vi "FCI_Lip_Gap.vi"(0 "Image":T4(plugin-control), 1 "Calibrated Image":T4, 2 "Search Direction Ref ROI":u32=2, 3 "Ref ROI":T5 {"Contours"."Type" items=["No Selection", "Point", "Line", "Rectangle", "Oval", "Polygon", "Freehand Region", "Annulus", "Unused2", "Unused3", "Broken Line", "Freehand Line", "Rotated Rectangle"]}, 4 "Meas ROI 1":T5 {"Contours"."Type" items=["No Selection", "Point", "Line", "Rectangle", "Oval", "Polygon", "Freehand Region", "Annulus", "Unused2", "Unused3", "Broken Line", "Freehand Line", "Rotated Rectangle"]}, 5 "error in (no error)":errorcluster, 6 "Line Options Ref ROI":T8={"Number of Lines"=1, "Type"=enum."Best Edge Rake", "Min. Score"=10.0, "Max. Score"=1000.0, "Orientation"=0.0, "Angle Range"=45.0, "Angle Tolerance"=1.0, "Step Size"=5, "Min. SNR (db)"=0.0, "Min. Points (%)"=25.0, "Hough Iterations"=5} {"Min. Points (%)" min=0.0 max=100.0; "Min. SNR (db)" min=0.0; "Max. Score" min=0.0 max=1024.0; "Min. Score" min=0.0 max=1024.0 step=1.0}, 7 "Edge Options Ref ROI":T6={"Edge Polarity"=0, "Kernel Size"=3, "Width"=3, "Minimum Edge Strength"=40.0, "Interpolation Type"=enum."Zero Order", "Data Processing Method"=enum."Average"} {"Edge Polarity" items=["All Edges", "Rising Edges", "Falling Edges"]; "Minimum Edge Strength" format="%.2f"; "Width" step=2; "Kernel Size" step=2}, 8 "Edge Options ROI 1":T6={"Edge Polarity"=0, "Kernel Size"=3, "Width"=3, "Minimum Edge Strength"=50.0, "Interpolation Type"=enum."Zero Order", "Data Processing Method"=enum."Average"} {"Edge Polarity" items=["All Edges", "Rising Edges", "Falling Edges"]; "Minimum Edge Strength" format="%.2f"; "Width" step=2; "Kernel Size" step=2}, 9 "Search Direction ROI 1":u16(ring) items=["Left To Right", "Right To Left", "Top To Bottom", "Bottom To Top"]) -> (13 "Overlay Arrow Lines":T1, 14 "Lip Gap Real World":sgl, 19 "error IO":errorcluster)   [LabVIEW 2019, in "Algorithm.lvclass"]
uses:
  FrameworkOverrides/Algorithm.lvclass
  <vilib>/vision/NI_Vision_Development_Module.lvlib
  <vilib>/vision/Measure.llb/Edge Polarity.ctl
  <vilib>/vision/Measure.llb/Edge Options.ctl
  <vilib>/vision/Measure.llb/Straight Edge Process.ctl
  <vilib>/vision/Measure.llb/Straight Edge Options.ctl
  <vilib>/vision/Image Controls.llb/IMAQ Image.ctl
panel:
  out "Second Overlay Line":T2
  out "First Overlay Line":T3
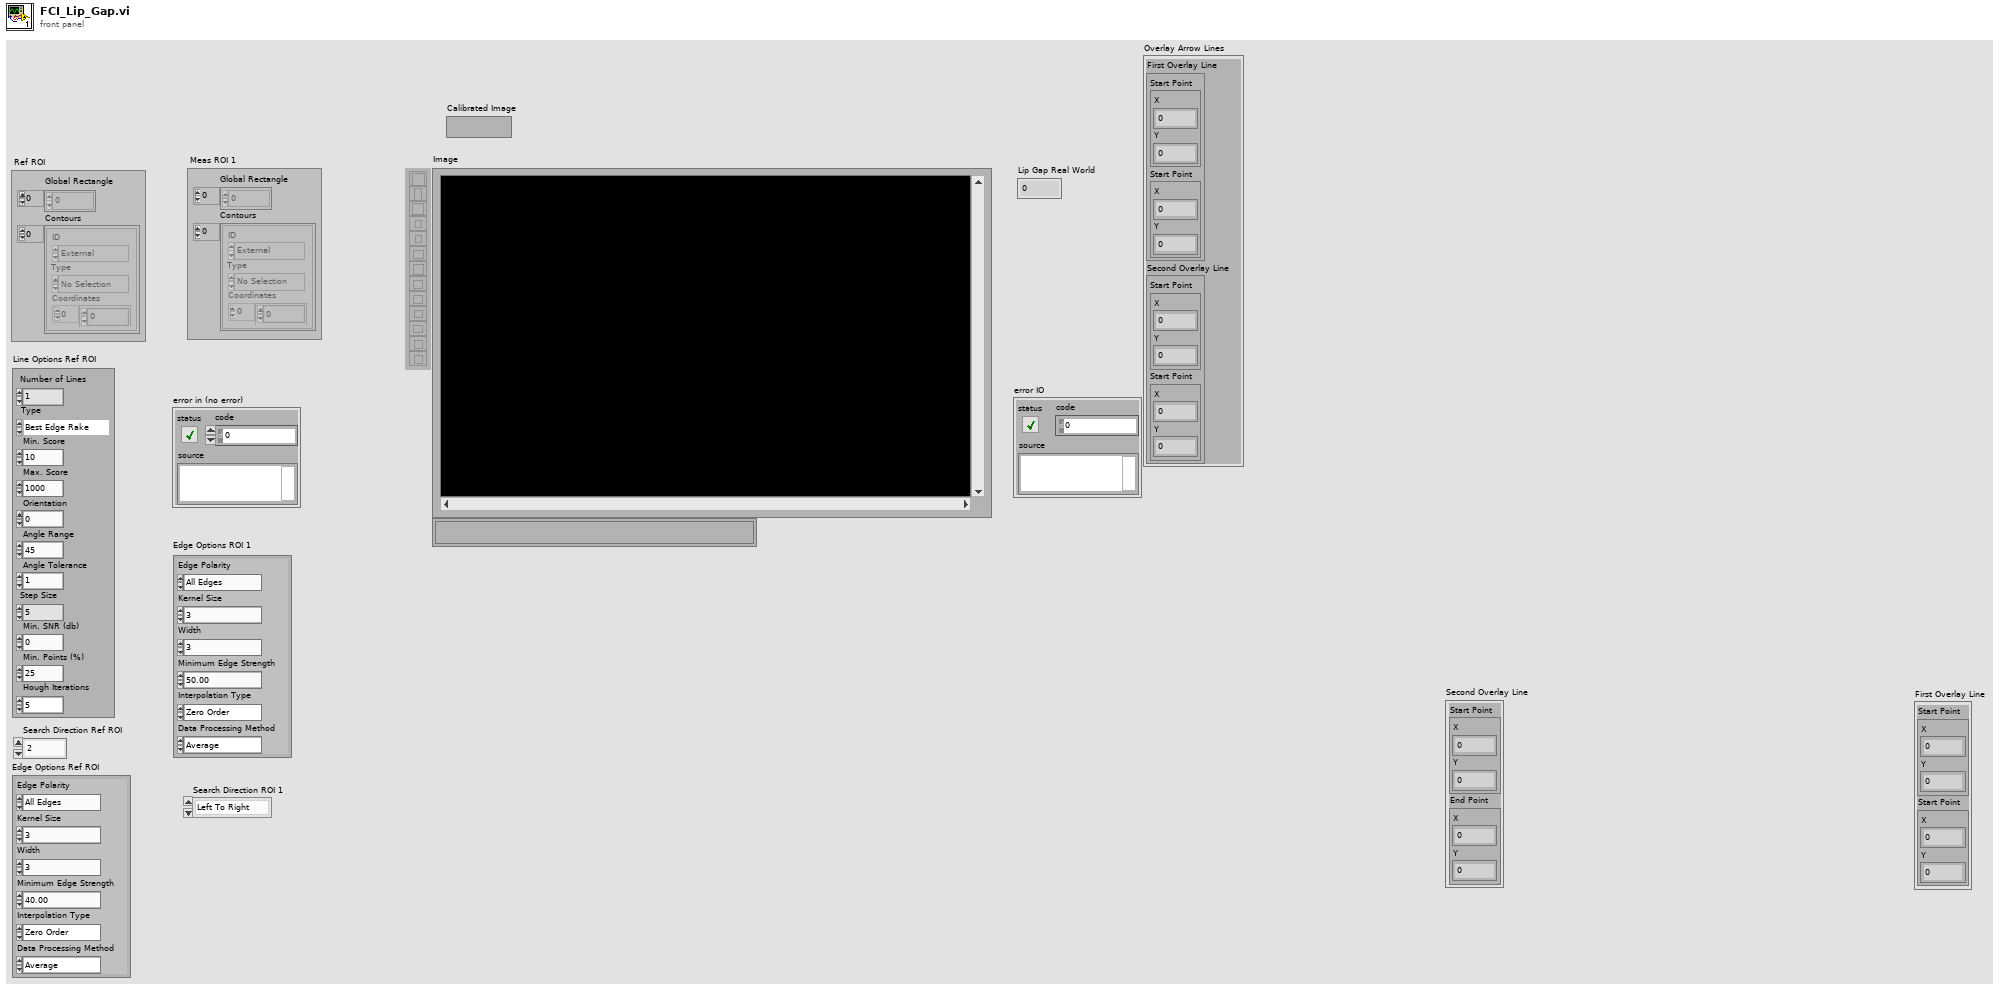
[diagram p1: front panel]
types:
  T1 = cluster{"First Overlay Line ":cluster{"Start Point":cluster{"X":sgl, "Y":sgl}, "Start Point":cluster{"X":sgl, "Y":sgl}}, "Second Overlay Line ":cluster{"Start Point":cluster{"X":sgl, "Y":sgl}, "Start Point":cluster{"X":sgl, "Y":sgl}}}
  T2 = cluster{"Start Point":cluster{"X":sgl, "Y":sgl}, "End Point":cluster{"X":sgl, "Y":sgl}}
  T3 = cluster{"Start Point":cluster{"X":sgl, "Y":sgl}, "Start Point":cluster{"X":sgl, "Y":sgl}}
  T4 = typedef "IMAQ Image.ctl" = refnum<image>
  T5 = typedef "ROI Descriptor" = cluster{"Global Rectangle":i32[], "Contours":cluster{"ID":enum32{"External", "Internal"}, "Type":u32, "Coordinates":i32[]}[]}
  T6 = typedef "Edge Options.ctl" = cluster{"Edge Polarity":T7, "Kernel Size":u32, "Width":u32, "Minimum Edge Strength":sgl, "Interpolation Type":enum32{"Zero Order", "Bilinear", "Quadratic", "Cubic", "Bilinear Fixed"}, "Data Processing Method":enum32{"Average", "Median"}}
  T7 = typedef "Edge Polarity.ctl" = u32
  T8 = typedef "Straight Edge Options.ctl" = cluster{"Number of Lines":i32, "Type":T9, "Min. Score":dbl, "Max. Score":dbl, "Orientation":dbl, "Angle Range":dbl, "Angle Tolerance":dbl, "Step Size":u32, "Min. SNR (db)":dbl, "Min. Points (%)":dbl, "Hough Iterations":i32}
  T9 = typedef "Straight Edge Process.ctl" = enum32{"First Edge Rake", "Best Edge Rake", "Hough Edge Rake", "First Edge Projection", "Best Edge Projection"}
  T10 = cluster{"Left":dbl, "Top":dbl, "Right":dbl, "Bottom":dbl, "Angle":dbl}
  T11 = enum16{"Get First Edge", "Get First + Last Edge", "Get All Edges", "Get Best Edge"}
  T12 = cluster{"Search Direction":u32, "Edge Options":T6, "Show Search Area":bool, "Show Search Lines":bool, "Show Edges Found":bool, "Show Result":bool, "Search Area Color":u32, "Search Lines Color":u32, "Edge Locations Color":u32, "Result Color":u32, "Overlay Group Name":string}
  T13 = cluster{"Point1 (Pixels)":cluster{"X":sgl, "Y":sgl}, "Point2 (Pixels)":cluster{"X":sgl, "Y":sgl}, "Point1 (Real-World)":cluster{"X":sgl, "Y":sgl}, "Point2 (Real-World)":cluster{"X":sgl, "Y":sgl}, "Angle (Pixel)":dbl, "Angle (Real-World)":dbl, "Score":dbl, "Straightness":dbl, "Average SNR (db)":dbl, "Calibration Valid":bool}[]
  T14 = cluster{"Point1 (Pixels)":cluster{"X":sgl, "Y":sgl}, "Point2 (Pixels)":cluster{"X":sgl, "Y":sgl}, "Point1 (Real-World)":cluster{"X":sgl, "Y":sgl}, "Point2 (Real-World)":cluster{"X":sgl, "Y":sgl}, "Angle (Pixel)":dbl, "Angle (Real-World)":dbl, "Score":dbl, "Straightness":dbl, "Average SNR (db)":dbl, "Calibration Valid":bool}
  T15 = typedef "Edge New.ctl" = cluster{"Location (Pixel)":cluster{"X":sgl, "Y":sgl}, "Location (Real-World)":cluster{"X":sgl, "Y":sgl}, "Distance (Pixel)":dbl, "Distance (Real-World)":dbl, "Strength":dbl, "Noise":dbl, "Rising?":bool}
  T16 = typedef "IMAQ Rectangle" = cluster{"Left":i32, "Top":i32, "Right":i32, "Bottom":i32, "Rotation":dbl}
  T17 = typedef "Search Line.ctl" = cluster{"Start Point":cluster{"X":sgl, "Y":sgl}, "End Point":cluster{"X":sgl, "Y":sgl}, "Edge Info":T15[], "Edge Map":dbl[], "Calibration Valid":bool}
  T18 = cluster{cluster{"X":sgl, "Y":sgl}, cluster{"X":sgl, "Y":sgl}}[]
  T19 = cluster{"Start Point":cluster{"X":sgl, "Y":sgl}, cluster{"X":sgl, "Y":sgl}}
  T20 = cluster{cluster{"X":sgl, "Y":sgl}, "End Point":cluster{"X":sgl, "Y":sgl}}
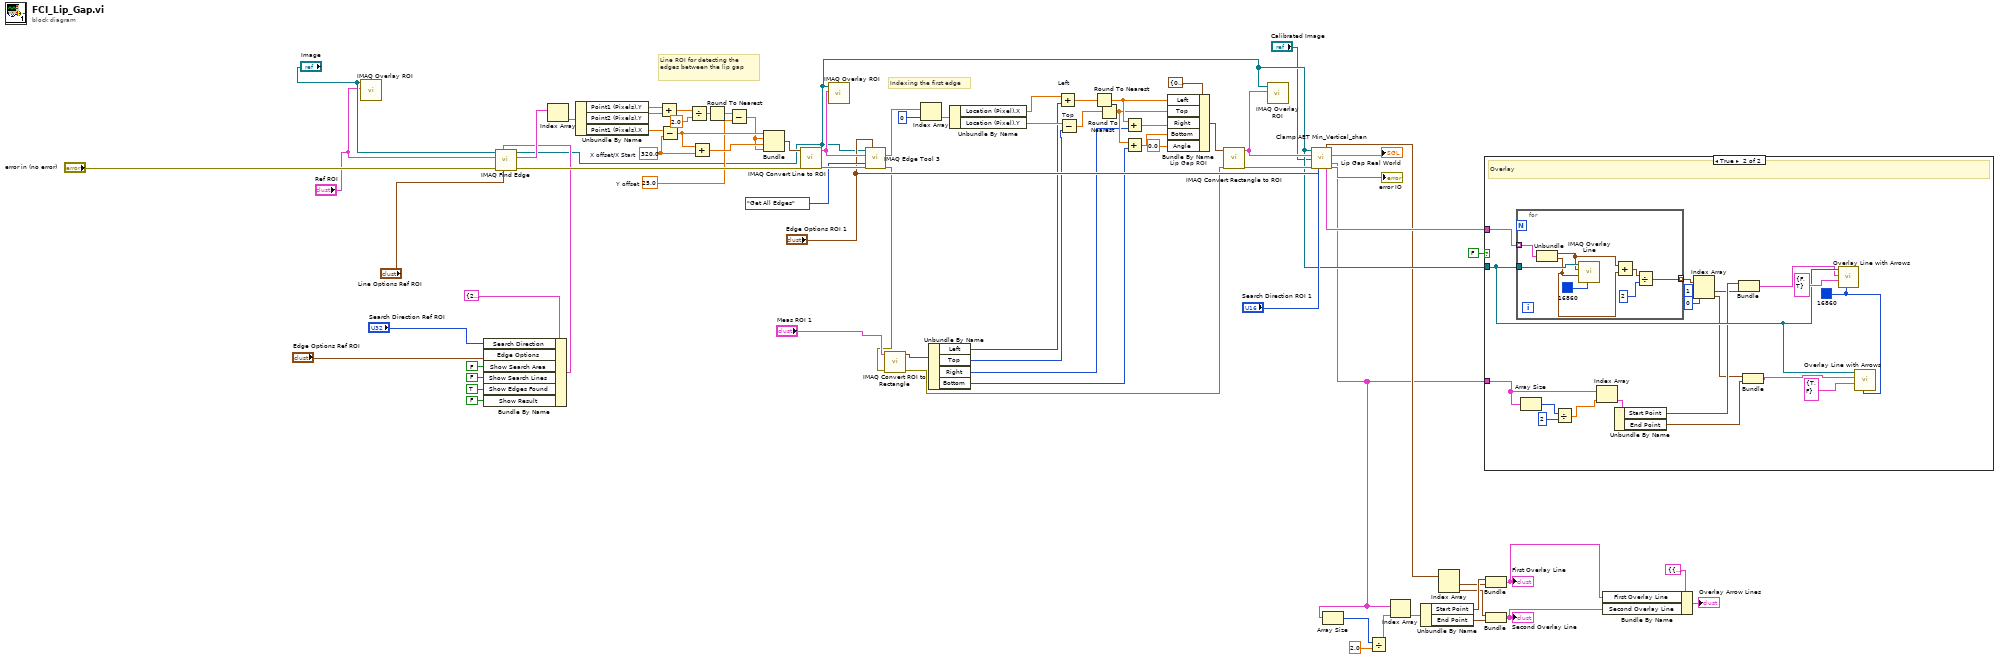
[diagram p0: block diagram]
diagram:
  w55 = sgl 25.0  # Y offset
  w63 = sgl 320.0  # X offset/X Start
  # "Indexing the first edge"
  # "Line ROI for detecting the edges between the lip gap"
  n1 = call "IMAQ Overlay ROI"("ROI Descriptor"="Ref ROI", "Image"="Image") -> ()  [unwired: 8 in, 2 out]
  n2 = Bundle By Name(cluster=T12 {"Search Direction"=2, "Edge Options"={"Edge Polarity"=0, "Kernel Size"=3, "Width"=3, "Minimum Edge Strength"=40.0, "Interpolation Type"=enum."Zero Order", "Data Processing Method"=enum."Average"}, "Show Search Area"=FALSE, "Show Search Lines"=FALSE, "Show Edges Found"=FALSE, "Show Result"=TRUE, "Search Area Color"=65280, "Search Lines Color"=255, "Edge Locations Color"=16776960, "Result Color"=16711680, "Overlay Group Name"=""} ("Options"), "Search Direction"="Search Direction Ref ROI", "Edge Options"="Edge Options Ref ROI", "Show Search Area"=FALSE, "Show Search Lines"=FALSE, "Show Edges Found"=TRUE, "Show Result"=FALSE) -> (w29:T12)
  n3 = call "IMAQ Find Edge"("Line Fit Options"="Line Options Ref ROI", "Options"=w29, "error in (no error)"="error in (no error)", "ROI Descriptor"="Ref ROI", "Image"="Image") -> ("error out"=w61:errorcluster, "Straight Edges"=w73:T13, "Image Out"=w27:T4)  [unwired: 3 in, 1 out]
  n4 = Index Array(array=w73) -> (element=w72:T14)  [unwired: 1 in]
  n5 = Unbundle By Name(w72) -> ("Point1 (Pixels).Y"=w71:sgl, "Point2 (Pixels).Y"=w70:sgl, "Point1 (Pixels).X"=w66:sgl)
  n6 = Add(x=w71, y=w70) -> (x+y=w69:sgl)
  n7 = Subtract(x=w66, y=w63) -> (x-y=w65:sgl)
  n8 = Divide(x=w69, y=sgl 2.0) -> (x/y=w67:sgl)
  n9 = Add(x=w65, y=w63) -> (x+y=w64:sgl)
  n10 = Round To Nearest(number=w67) -> (nearest integer value=w56:sgl)
  n11 = Subtract(x=w56, y=w55) -> (x-y=w57:sgl)
  n12 = Bundle(w65, w57, w64, w57) -> (w62:cluster{sgl, sgl, sgl, sgl})  [unwired: 1 in]
  n13 = call "IMAQ Convert Line to ROI"("error in (no error)"=w61, "Line"=w62) -> ("error out"=w60:errorcluster, "ROI Descriptor"=w58:T5)  [unwired: 7 in]
  n14 = call "IMAQ Overlay ROI"("ROI Descriptor"=w58, "Image"=w27) -> ()  [unwired: 8 in, 2 out]
  n15 = call "IMAQ Edge Tool 3"("Image"=w27, "Edge Options"="Edge Options ROI 1", "ROI Descriptor"=w58, "Process"=T11."Get All Edges", "error in (no error)"=w60) -> ("Edge Information"=w54:T15[], "error out"=w20:errorcluster)  [unwired: 6 in, 3 out]
  n16 = call "IMAQ Convert ROI to Rectangle"("error in (no error)"=w20, "ROI Descriptor"="Meas ROI 1") -> ("error out"=w19:errorcluster, "Rectangle"=w25:T16)  [unwired: 7 in]
  n17 = Index Array(array=w54, index=0) -> (element=w53:T15)
  n18 = Unbundle By Name(w25) -> ("Left"=w24:i32, "Top"=w23:i32, "Right"=w22:i32, "Bottom"=w21:i32)
  n19 = Unbundle By Name(w53) -> ("Location (Pixel).X"=w49:sgl, "Location (Pixel).Y"=w48:sgl)
  n20 = Add "Left"(x=w49, y=w24) -> (x+y=w47:sgl)
  n21 = Subtract "Top"(x=w48, y=w23) -> (x-y=w46:sgl)
  n22 = Round To Nearest(number=w47) -> (nearest integer value=w44:sgl)
  n23 = Round To Nearest(number=w46) -> (nearest integer value=w42:sgl)
  n24 = Add(x=w44, y=w22) -> (x+y=w43:sgl)
  n25 = Add(x=w42, y=w21) -> (x+y=w41:sgl)
  n26 = Bundle By Name "Lip Gap ROI"(cluster=T10 {"Left"=0.0, "Top"=0.0, "Right"=0.0, "Bottom"=0.0, "Angle"=0.0} ("input cluster"), "Left"=w44, "Top"=w42, "Right"=w43, "Bottom"=w41, "Angle"=0.0) -> (w45:T10)
  n27 = call "IMAQ Convert Rectangle to ROI"("error in (no error)"=w19, "Rectangle"=w45) -> ("error out"=w40:errorcluster, "ROI Descriptor"=w39:T5)  [unwired: 7 in]
  n28 = call "IMAQ Overlay ROI"("ROI Descriptor"=w39, "Image"=w27) -> ()  [unwired: 8 in, 2 out]
  n29 = call "Clamp AET Min_Vertical_shan.vi"("Image"=w27, "Scanning axis"="Search Direction ROI 1", "ROI Descriptor"=w39, "Calibrated Image"="Calibrated Image", "error in (no error)"=w40, "Edge Options"="Edge Options ROI 1") -> ("Edge Coordinates"=w3:cluster{"X":sgl, "Y":sgl}[], "Distance"=→"Lip Gap Real World":sgl, "Search Lines"=w2:T17[], "Perpendicular Lines"=w76:T18, "error out"=→"error IO":errorcluster)  [unwired: 3 in, 2 out]
  n30 = Array Size(array=w2) -> (size(s)=w5:i32)
  n31 = Divide(x=w5, y=2.0) -> (x/y=w4:dbl)
  n32 = Index Array(array=w2, index=w4) -> (element=w14:T17)
  n33 = Unbundle By Name(w14) -> ("Start Point"=w13:cluster{"X":sgl, "Y":sgl}, "End Point"=w10:cluster{"X":sgl, "Y":sgl})
  n34 = Index Array(array=w3) -> (element #1=w12:cluster{"X":sgl, "Y":sgl}, element #2=w11:cluster{"X":sgl, "Y":sgl})  [unwired: 2 in]
  n35 = case shown="True" FALSE {
    tunnel: w76 -> [_ w96]
    tunnel: w27 -> [_ w88]
    tunnel: w2 -> [_ w93]
    frame False {
    }
    frame True {
      w80 = u32 16860 ("Color")
      # "Overlay"
      n36 = for {
        tunnel: w96 -> [w104] mode=indexing
        tunnel: w88 -> [w103]
        tunnel: [w97] -> w87 mode=indexing
        n37 = Unbundle(w104) -> (w101:cluster{"X":sgl, "Y":sgl}, w100:cluster{"X":sgl, "Y":sgl})
        n38 = call "IMAQ Overlay Line"("Color"=u32 16860, "End Point"=w100, "Start Point"=w101, "Image"=w103) -> ()  [unwired: 6 in, 2 out]
        n39 = Add(x=w101, y=w100) -> (x+y=w99:cluster{"X":sgl, "Y":sgl})
        n40 = Divide(x=w99, y=2) -> (x/y=w97:cluster{"X":sgl, "Y":sgl})
      }
      n41 = Array Size(array=w93) -> (size(s)=w95:i32)
      n42 = Divide(x=w95, y=2) -> (x/y=w92:dbl)
      n43 = Index Array(array=w93, index=w92) -> (element=w91:T17)
      n44 = Unbundle By Name(w91) -> ("Start Point"=w86:cluster{"X":sgl, "Y":sgl}, "End Point"=w83:cluster{"X":sgl, "Y":sgl})
      n45 = Index Array(array=w87, index #1=1 ("index"), index #2=0 ("index")) -> (element #1=w85:cluster{"X":sgl, "Y":sgl}, element #2=w84:cluster{"X":sgl, "Y":sgl})
      n46 = Bundle("Start Point"=w86, w85) -> (w82:T19)  [unwired: 1 in]
      n47 = Bundle(w84, "End Point"=w83) -> (w81:T20)  [unwired: 1 in]
      n48 = call <vilib>:"Overlay Line with Arrows.vi"("Color"=w80, "Arrows"=cluster{"Start point":bool, "End point":bool} {"Start point"=FALSE, "End point"=TRUE}, "Line Coordinates"=w82, "Image In"=w88) -> ()  [unwired: 6 in, 2 out]
      n49 = call <vilib>:"Overlay Line with Arrows.vi"("Color"=w80, "Arrows"=cluster{"Start point":bool, "End point":bool} {"Start point"=TRUE, "End point"=FALSE}, "Line Coordinates"=w81, "Image In"=w88) -> ()  [unwired: 6 in, 2 out]
    }
  }
  n50 = Bundle("Start Point"=w13, w12) -> (w8:T19)  [unwired: 1 in]
  "First Overlay Line" <- w8
  n51 = Bundle(w11, "End Point"=w10) -> (w7:T20)  [unwired: 1 in]
  "Second Overlay Line" <- w7
  n52 = Bundle By Name(cluster=T1 {"First Overlay Line "={"Start Point"={"X"=0.0, "Y"=0.0}, "Start Point"={"X"=0.0, "Y"=0.0}}, "Second Overlay Line "={"Start Point"={"X"=0.0, "Y"=0.0}, "Start Point"={"X"=0.0, "Y"=0.0}}}, "First Overlay Line"=w8, "Second Overlay Line"=w7) -> (→"Overlay Arrow Lines":T1)
